vi "Reverse Data Set.vi"(9 "Pos to Start Scan":i32, 10 "Scan Data Array in":u8[][](array[numeric]), 11 "Array Size":i32) -> (2 "Reversed Array out":u8[][](array[numeric]))   [LabVIEW 2015, in "Tool Module.lvlib"]
doc: "<b>Note:</b> This VI was modified by the <b>Validate DQMH Module</b> tool to turn off automatic error handling."
uses:
  Tool Module.lvlib
  Tool Config/Tool Cfg.lvlib
panel:
  out "Axial Pos Array":dbl[](array[numeric]) format="%#.4g"
  out "Axial Positions":dbl[](graph)
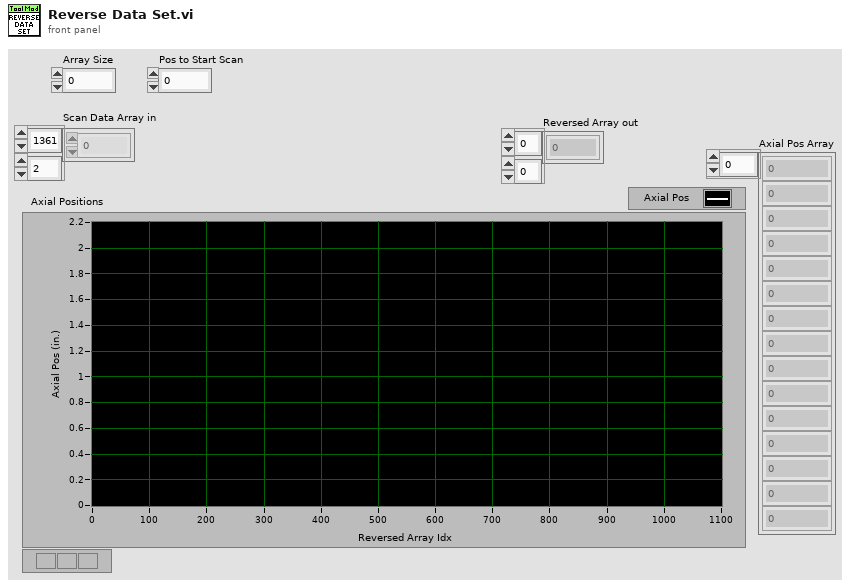
[diagram p1: front panel]
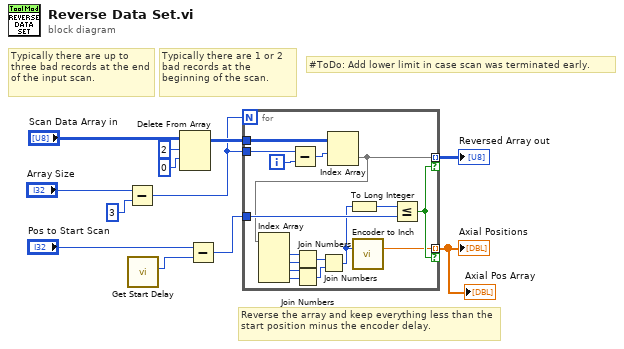
[diagram p0: block diagram]
diagram:
  # "#ToDo: Add lower limit in case scan was terminated early."
  # "Typically there are 1 or 2 bad records at the beginning of the scan."
  # "Typically there are up to three bad records at the end of the input scan."
  # "Reverse the array and keep everything less than the start position minus the encoder delay."
  n1 = Subtract(x="Array Size", y=3 ("x")) -> (x-y=w6:i32)
  n2 = call "Get Start Delay.vi"() -> ("Encoder out"=w1:i32)  [unwired: 10 in, 1 out]
  n3 = Delete From Array(array="Scan Data Array in", length=2, index (row)=0) -> (array with subset deleted=w7:u8[][])  [unwired: 1 in, 1 out]
  n4 = Subtract(x="Pos to Start Scan", y=w1) -> (x-y=w3:i32)
  n5 = for {
    N: w6 -> [_]
    tunnel: w7 -> [w28]
    tunnel: w6 -> [w27]
    tunnel: [w15] -> w4 mode=indexing if=w16
    tunnel: [w13] -> w5 mode=indexing if=w16
    tunnel: w3 -> [w18]
    i -> [w26]
    n6 = Subtract(x=w27, y=w26) -> (x-y=w25:i32)
    n7 = Index Array(array=w28, index (row)=w25) -> (element=w15:u8[])  [unwired: 1 in]
    n8 = Index Array(array=w15) -> (element #1=w20:u8, element #2=w19:u8, element #3=w21:u8, element #4=w22:u8)  [unwired: 4 in]
    n9 = Join Numbers(hi=w20, lo=w19) -> ((hi.lo)=w23:u16)
    n10 = Join Numbers(hi=w21, lo=w22) -> ((hi.lo)=w24:u16)
    n11 = Join Numbers(hi=w23, lo=w24) -> ((hi.lo)=w14:u32)
    n12 = To Long Integer(number=w14) -> (32bit integer=w17:i32)
    n13 = call "Encoder to Inch.vi"("Encoder in"=w14) -> ("Encoder out(in)"=w13:dbl)  [unwired: 14 in]
    n14 = Less Or Equal?(x=w17, y=w18) -> (x <= y?=w16:bool)
  }
  "Axial Positions" <- w5
  "Reversed Array out" <- w4
  "Axial Pos Array" <- w5
